vi "Actor Core.vi"(8 "error in":errorcluster, 11 "Measure-Pulse in":refnum<class "Monitor-Pulse.lvclass">) -> (0 "error out":errorcluster, 3 "Actor out":refnum<class "Actor.lvclass">)   [LabVIEW 2016, in "Monitor-Pulse.lvclass"]
doc: "(<B>Filename</B>: Actor Framework.lvlib:Actor.lvclass:Actor Core.vi)\n\nReceives messages to the actor, reacts to them, and initiates any error handling that may shut the actor down.\n\nDescendant classes may override this VI to append parallel tasks for the actor to complete while it handles messages. Overrides use the Call Parent Method node."
uses:
  Monitor-Pulse.lvclass
  D:/github/Measure_core/Da Base/Da Base.lvclass
  D:/Program Files/National Instruments/LabVIEW 2016/vi.lib/ActorFramework/Actor/Actor.lvclass
  <vilib>/ActorFramework/Actor/Actor.lvclass
  NHMFL_Core/Libraries/Queued Listbox/Queued Listbox.xctl
  Monitor-Pulse.lvclass/Monitor-Pulse.ctl
  Measure_core/Da Base/Da Base.lvclass/Da Base.ctl
  <vilib>/ActorFramework/Actor/Actor.lvclass/Actor.ctl
  <vilib>/ActorFramework/Message Enqueuer/Message Enqueuer.lvclass/Message Enqueuer.ctl
  Measure_core/Controllers/Application Controller Messages/Pulse Acquired Result/Pulse Acquired Result.lvclass
  D:/github/Measure_core/Da Base Messages/Result Reply Msg/Result Reply Msg.lvclass
  Monitor-Pulse Messages/Start Pulse Measurements Msg/Start Measurements Command Msg.lvclass/Start Measurements Command Msg.ctl
  <vilib>/Utility/sysdir.llb/System Directory Type.ctl
  Measure_core/Da Base Messages/Save Configuration Msg/Save Configuration Msg.lvclass/Save Configuration Msg.ctl
  Measure_core/Da Base Messages/Open Item Msg/Open Item Msg.lvclass/Open Item Msg.ctl
  Measure_core/Plots/Plot types.ctl
  Measure_core/Controllers/Application Controller Messages/Open Waveform File Plot Msg/Open Waveform File Plot Msg.lvclass/Open Waveform File Plot Msg.ctl
  Monitor-Pulse Messages/Stop Measurements Command Msg/Stop Measurements Command Msg.lvclass/Stop Measurements Command Msg.ctl
  Measure_core/da Base/Read stop event.vi
  Measure_core/da Base/Read Open item event.vi
  <vilib>/ActorFramework/Message Enqueuer/Init from Existing Queue.vi
  <vilib>/ActorFramework/Message Enqueuer/Enqueue.vi
  <vilib>/ActorFramework/Stop Msg/Stop Msg.lvclass
  D:/Program Files/National Instruments/LabVIEW 2016/vi.lib/ActorFramework/Message/Message.lvclass
  Monitor-Pulse Messages/Start Pulse Measurements Msg/Start Measurements Command Msg.lvclass
  Measure_core/Da Base Messages/Save Configuration Msg/Save Configuration Msg.lvclass
  Measure_core/Da Base Messages/Open Item Msg/Open Item Msg.lvclass
  Measure_core/Controllers/Application Controller Messages/Open Waveform File Plot Msg/Open Waveform File Plot Msg.lvclass
  Monitor-Pulse Messages/Stop Measurements Command Msg/Stop Measurements Command Msg.lvclass
  <vilib>/ActorFramework/Message Priority Queue/Priority Enqueue.vi
  Measure_core/Controllers/Application Controller/Application Controller.lvclass
  <vilib>/ActorFramework/Message Enqueuer/Message Enqueuer.lvclass
  Measure_core/da Base Messages/Restore Configuration Msg/Restore Configuration Msg.lvclass
panel:
  in  "Full XY Plot":bool
  out "Monitor file":path caption="Current\nFile"
  in  "View Waveform":bool
  out "PEAK FIELD":dbl format="%#.2g"
  in  "Exit":bool
  in  "Monitor configuration":bool
  in  "Pulse configuration":bool
  in  "Refresh Button":bool
  out "Pulse file":path caption="Last\nFile"
  in  "Write cfg":bool
  in  "Read cfg":bool
  in  "View XY Plot":bool
  out "Monitor Running":bool
  out "Armed":bool
  in  "Arm":bool
  in  "Stop monitor":bool
  in  "Start monitor":bool
  in  "Monitor":string[](xcontrol)
  in  "Process":string[](xcontrol)
  in  "Acquire Pulse":string[](xcontrol)
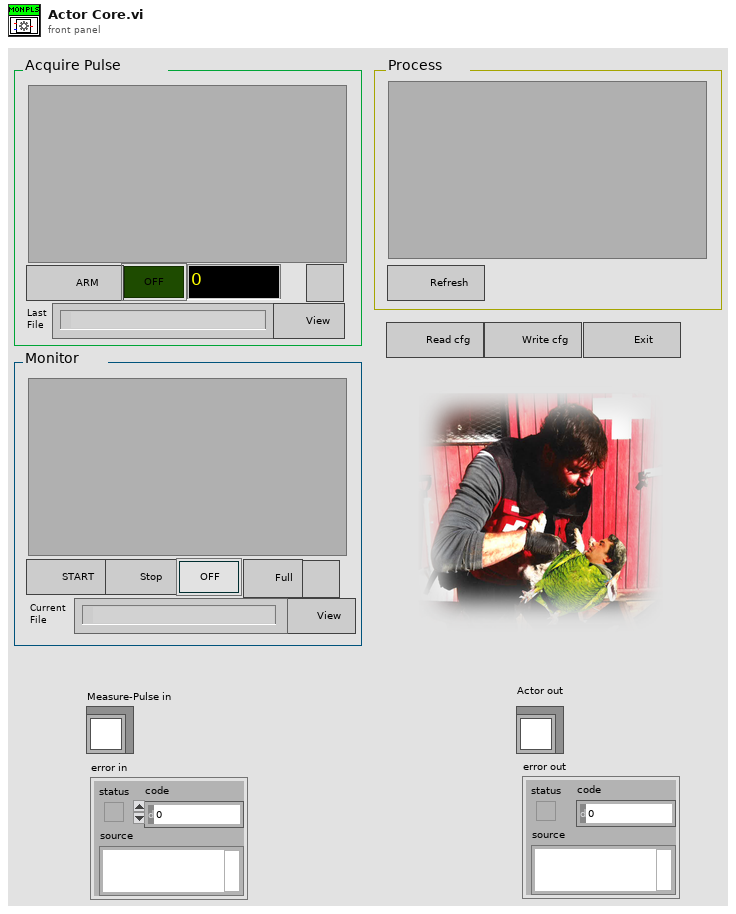
[diagram p1: front panel]
types:
  T1 = typedef "Plot types.ctl" = enum16{"Waveform Plot", "XY Plot", "Full XY"}
  T2 = typedef "System Directory Type.ctl" = i32
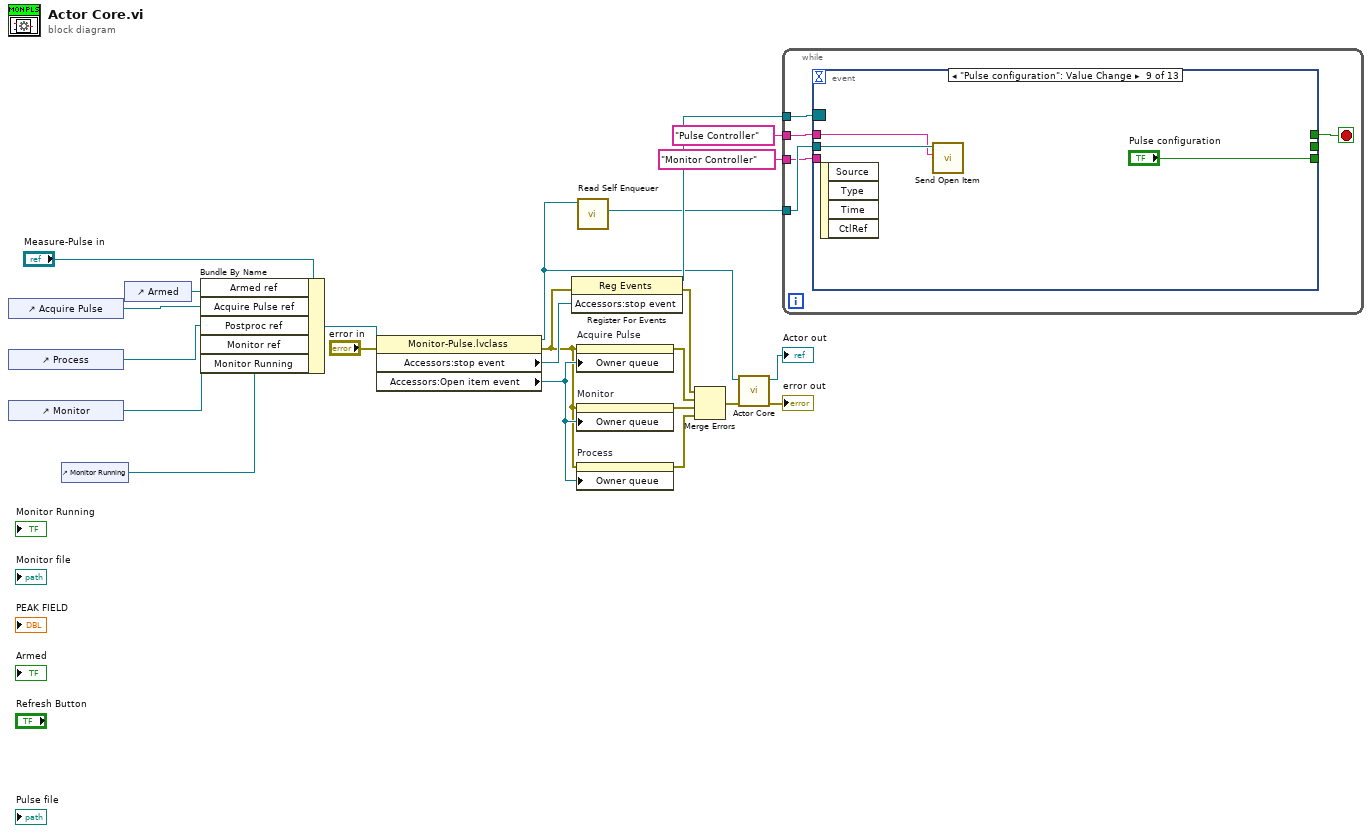
[diagram p0: block diagram]
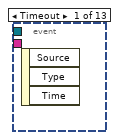
[diagram p2: hidden frame]
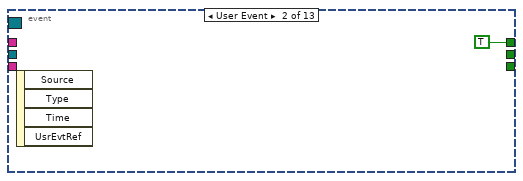
[diagram p3: hidden frame]
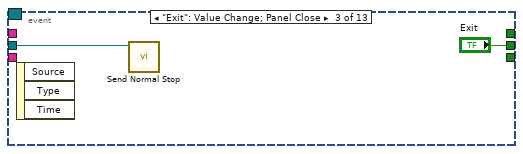
[diagram p4: hidden frame]
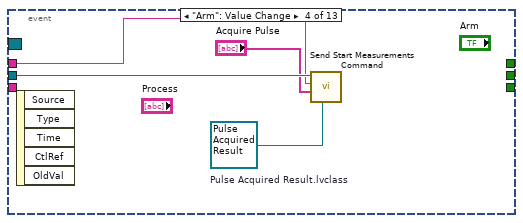
[diagram p5: hidden frame]
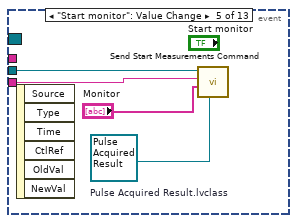
[diagram p6: hidden frame]
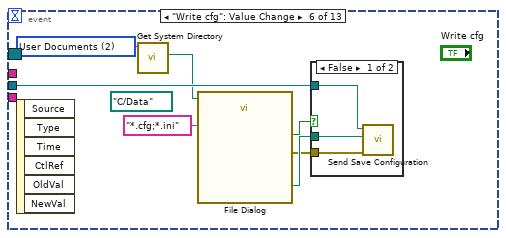
[diagram p7: hidden frame]
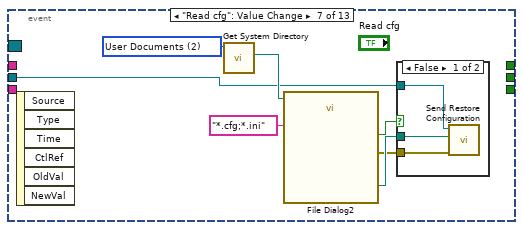
[diagram p9: hidden frame]
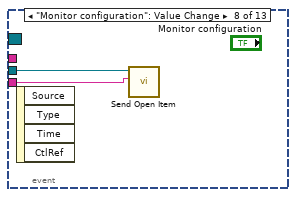
[diagram p11: hidden frame]
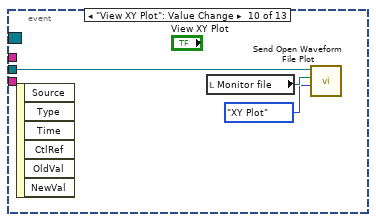
[diagram p12: hidden frame]
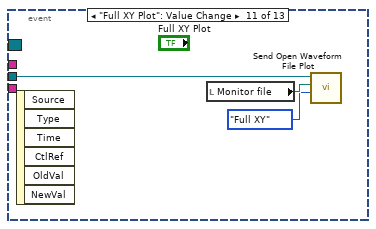
[diagram p13: hidden frame]
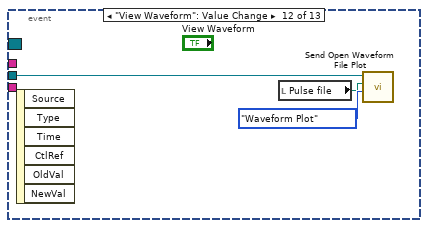
[diagram p14: hidden frame]
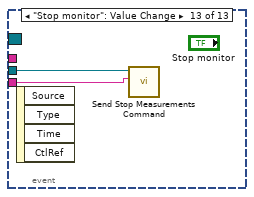
[diagram p15: hidden frame]
diagram:
  n1 = control-ref of="Acquire Pulse"() -> (w6:refnum<vi>)
  n2 = control-ref of="Process"() -> (w5:refnum<vi>)
  n3 = control-ref of="Monitor"() -> (w2:refnum<vi>)
  n4 = control-ref of="Monitor Running"() -> (w1:refnum<vi>)
  n5 = control-ref of="Armed"() -> (w7:refnum<vi>)
  n6 = Bundle By Name(cluster="Measure-Pulse in", "Armed ref"=w7, "Acquire Pulse ref"=w6, "Postproc ref"=w5, "Monitor ref"=w2, "Monitor Running"=w1) -> (w8:refnum<class "Monitor-Pulse.lvclass">)
  n7 = property class="Monitor-Pulse.lvclass"(reference=w8, error in="error in") -> (reference out=w10:refnum<class "Monitor-Pulse.lvclass">, error out=w14:errorcluster, "Accessors:stop event"=w20:refnum<user-event>, "Accessors:Open item event"=w18:refnum<user-event>)
  n8 = register-events(error in=w14, w20) -> (reference out=w19:refnum<event-registration>, error out=w13:errorcluster)  [unwired: 1 in]
  n9 = property on="Acquire Pulse" class="Queued Listbox (strict)"(error in=w14, "Owner queue"=w18) -> (error out=w17:errorcluster)  [unwired: 1 in, 1 out]
  n10 = property on="Monitor" class="Queued Listbox (strict)"(error in=w14, "Owner queue"=w18) -> (error out=w16:errorcluster)  [unwired: 1 in, 1 out]
  n11 = property on="Process" class="Queued Listbox (strict)"(error in=w14, "Owner queue"=w18) -> (error out=w15:errorcluster)  [unwired: 1 in, 1 out]
  n12 = call <vilib>:"Read Self Enqueuer.vi"("Actor"=w10) -> ("Self Enqueuer"=w9:refnum<class "Message Enqueuer.lvclass">)  [unwired: 10 in]
  n13 = Merge Errors(w13, w17, w16, w15) -> (w11:errorcluster)
  n14 = call-parent "Actor Core.vi"("error in"=w11, "Measure Object in"=w10) -> ("error out"=→"error out":errorcluster, "Actor out"=→"Actor out":refnum<class "Actor.lvclass">)  [unwired: 8 in]
  n15 = while {
    tunnel: w19 -> [w28]
    tunnel: w9 -> [w26]
    tunnel: "Monitor Controller" ("Controller name") -> [w25]
    tunnel: "Pulse Controller" ("Item name") -> [w24]
    stop <- w27 stop-if-true
    n16 = event shown="[8] \"Pulse configuration\": Value Change" {
      selector: w28 -> [_ _ _ _ _ _ _ _ _ _ _ _ _]
      dyn-events: _ -> [_ _ _ _ _ _ _ _ _ _ _ _ _]
      timeout: _ -> [_ _ _ _ _ _ _ _ _ _ _ _ _]
      tunnel: [_ TRUE _ _ _ _ _ _ _ _ _ _ _] -> w27
      tunnel: w26 -> [_ _ w30 w35 w38 w43 w51 w61 w63 w67 w70 w72 w75]
      tunnel: [_ _ _ _ _ _ _ _ "Pulse configuration" _ _ _ _] -> _
      tunnel: [_ _ "Exit" _ _ _ _ _ _ _ _ _ _] -> _
      tunnel: w25 -> [_ _ _ _ w37 _ _ w60 _ _ _ _ w74]
      tunnel: w24 -> [_ _ _ w33 _ _ _ _ w62 _ _ _ _]
      event Timeout {
        n17 = event-data() -> ()  [unwired: 1 in, 3 out]
      }
      event User Event {
        n18 = event-data() -> ()  [unwired: 1 in, 4 out]
      }
      event "Exit": Value Change; Panel Close {
        n19 = event-data() -> ()  [unwired: 1 in, 3 out]
        n20 = call <vilib>:"Send Normal Stop.vi"("Message Enqueuer"=w30) -> ()  [unwired: 10 in, 1 out]
      }
      event "Arm": Value Change {
        w32 = refnum<class "Pulse Acquired Result.lvclass"> refnum  # Pulse Acquired Result.lvclass
        n21 = event-data() -> ()  [unwired: 1 in, 5 out]
        n22 = call "Send Start Measurements Command.vi"("Reply to me"=w32, "Objects"="Acquire Pulse", "Controller name"=w33, "Message Enqueuer"=w35) -> ()  [unwired: 6 in, 2 out]
      }
      event "Start monitor": Value Change {
        w36 = refnum<class "Pulse Acquired Result.lvclass"> refnum  # Pulse Acquired Result.lvclass
        n23 = event-data() -> ()  [unwired: 1 in, 6 out]
        n24 = call "Send Start Measurements Command.vi"("Reply to me"=w36, "Objects"="Monitor", "Controller name"=w37, "Message Enqueuer"=w38) -> ()  [unwired: 6 in, 2 out]
      }
      event "Write cfg": Value Change {
        w41 = T2 2 items=["User Home"=0, "User Desktop"=1, "User Documents"=2, "User Application Data"=3, "User Preferences"=4, "User Temporary"=5, "Public Documents"=6, "Public Application Data"=7, "Public Preferences"=8, "Public Cache"=13, "System Core Libraries"=9, "System Installed Libraries"=10, "Application Files"=11, "Boot Volume Root"=12] ("system directory type")
        (unwired) path "C:/Data" ("start path")
        n25 = event-data() -> ()  [unwired: 1 in, 6 out]
        n26 = call <vilib>:"Get System Directory.vi"("system directory type"=w41) -> ("system directory"=w40:path)  [unwired: 10 in]
        n27 = call "File Dialog"("start path"=w40, "pattern (all files)"="*.cfg;*.ini") -> ("selected path"=w45:path, "cancelled"=w46:bool, "error out"=w42:errorcluster)  [unwired: 10 in, 1 out]
        n28 = case shown="False" w46 {
          tunnel: w45 -> [w47 _]
          tunnel: w43 -> [w49 _]
          tunnel: w42 -> [w48 _]
          frame False {
            n29 = call "Send Save Configuration.vi"("error in (no error)"=w48, "File path"=w47, "Message Enqueuer"=w49) -> ()  [unwired: 7 in, 2 out]
          }
          frame True {
          }
        }
      }
      event "Read cfg": Value Change {
        w53 = T2 2 items=["User Home"=0, "User Desktop"=1, "User Documents"=2, "User Application Data"=3, "User Preferences"=4, "User Temporary"=5, "Public Documents"=6, "Public Application Data"=7, "Public Preferences"=8, "Public Cache"=13, "System Core Libraries"=9, "System Installed Libraries"=10, "Application Files"=11, "Boot Volume Root"=12] ("system directory type")
        n30 = event-data() -> ()  [unwired: 1 in, 6 out]
        n31 = call <vilib>:"Get System Directory.vi"("system directory type"=w53) -> ("system directory"=w52:path)  [unwired: 10 in]
        n32 = call "File Dialog2"("start path"=w52, "pattern (all files)"="*.cfg;*.ini") -> ("selected path"=w56:path, "cancelled"=w50:bool, "error out"=w54:errorcluster)  [unwired: 10 in, 1 out]
        n33 = case shown="False" w50 {
          tunnel: w56 -> [w57 _]
          tunnel: w51 -> [w59 _]
          tunnel: w54 -> [w58 _]
          frame False {
            n34 = call "Send Restore Configuration.vi"("error in (no error)"=w58, "File path"=w57, "Message Enqueuer"=w59) -> ()  [unwired: 7 in, 2 out]
          }
          frame True {
          }
        }
      }
      event "Monitor configuration": Value Change {
        n35 = event-data() -> ()  [unwired: 1 in, 4 out]
        n36 = call "Send Open Item.vi"("Item name"=w60, "Message Enqueuer"=w61) -> ()  [unwired: 8 in, 2 out]
      }
      event "Pulse configuration": Value Change {
        n37 = event-data() -> ()  [unwired: 1 in, 4 out]
        n38 = call "Send Open Item.vi"("Item name"=w62, "Message Enqueuer"=w63) -> ()  [unwired: 8 in, 2 out]
      }
      event "View XY Plot": Value Change {
        n39 = event-data() -> ()  [unwired: 1 in, 6 out]
        n40 = local read "Monitor file"() -> (w66:path)
        n41 = call "Send Open Waveform File Plot.vi"("Plot type"=Plot_types."XY Plot", "File Path Control"=w66, "Message Enqueuer"=w67) -> ()  [unwired: 7 in, 2 out]
      }
      event "Full XY Plot": Value Change {
        n42 = event-data() -> ()  [unwired: 1 in, 6 out]
        n43 = local read "Monitor file"() -> (w69:path)
        n44 = call "Send Open Waveform File Plot.vi"("Plot type"=Plot_types."Full XY", "File Path Control"=w69, "Message Enqueuer"=w70) -> ()  [unwired: 7 in, 2 out]
      }
      event "View Waveform": Value Change {
        n45 = event-data() -> ()  [unwired: 1 in, 6 out]
        n46 = local read "Pulse file"() -> (w71:path)
        n47 = call "Send Open Waveform File Plot.vi"("Plot type"=Plot_types."Waveform Plot", "File Path Control"=w71, "Message Enqueuer"=w72) -> ()  [unwired: 7 in, 2 out]
      }
      event "Stop monitor": Value Change {
        n48 = event-data() -> ()  [unwired: 1 in, 4 out]
        n49 = call "Send Stop Measurements Command.vi"("Measurement Controller"=w74, "Message Enqueuer"=w75) -> ()  [unwired: 8 in, 2 out]
      }
    }
  }
